vi "MSCOMM.vi"(0 "端口号":string="COM7", 1 "MSComm":refnum<k7>(container), 5 "Send Delay(ms)":string="100", 7 "Send Data":string="AT\r\n", 9 "Data Return":string="OK", 11 "cycle times":string="3") -> (4 "result":bool, 8 "Rec Data":string, 10 "Para":string)   [LabVIEW 2013]
panel:
  out "字符串":string
  out "接收数据长度字节数目":i32
  out "PortOpen":bool
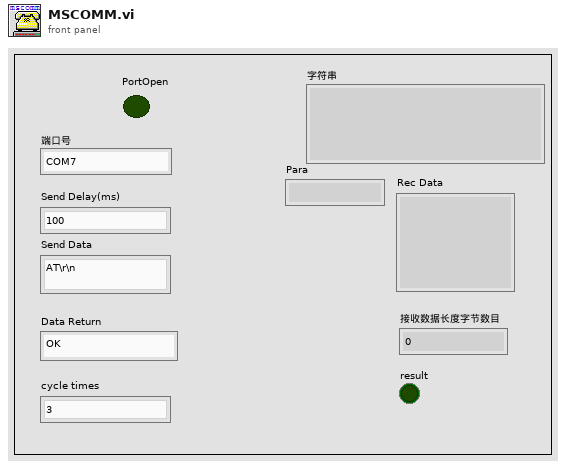
[diagram p1: front panel]
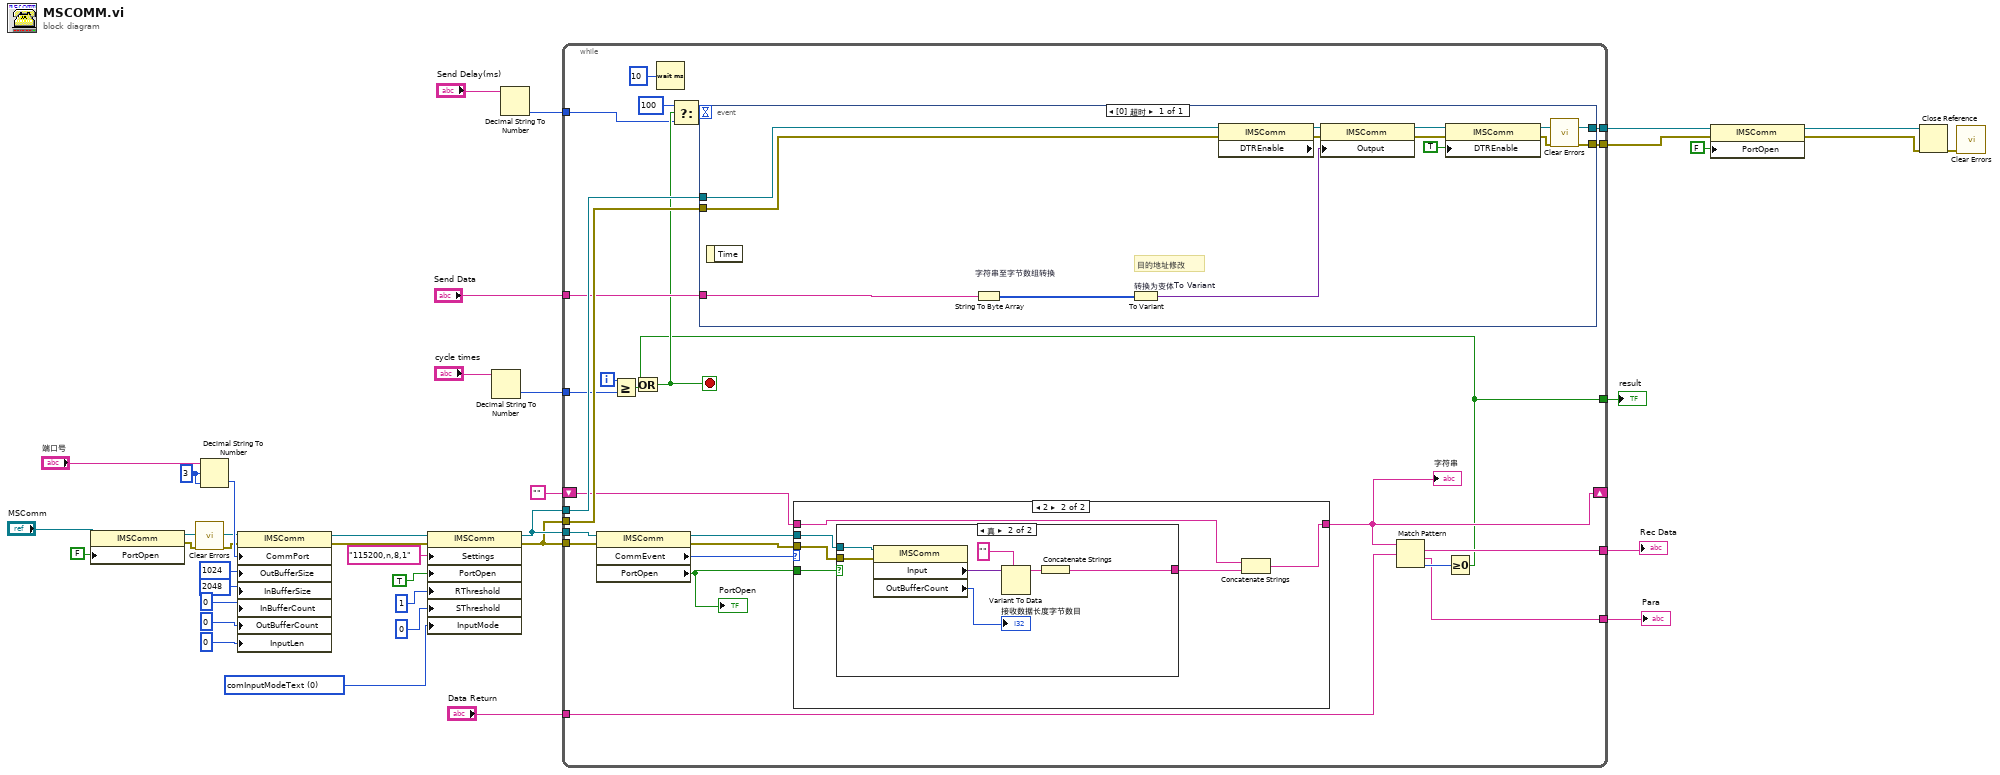
[diagram p0: block diagram]
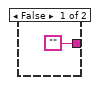
[diagram p3: hidden frame]
diagram:
  w8 = 3 ("偏移量")
  w26 = 0 items=["comInputModeText", "comInputModeBinary"] ("InputMode")
  n1 = property class="IMSComm"(reference="MSComm", "PortOpen"=FALSE) -> (reference out=w6:refnum<k7>, error out=w5:errorcluster)  [unwired: 1 in]
  n2 = call <vilib>:"Clear Errors.vi"("error in (no error)"=w5) -> ("error out"=w4:errorcluster)  [unwired: 6 in]
  n3 = Decimal String To Number(string="端口号", offset=w8, default (0L)=w8) -> (number=w17:i32)  [unwired: 1 out]
  n4 = property class="IMSComm"(reference=w6, error in=w4, "CommPort"=w17, "OutBufferSize"=i16 1024, "InBufferSize"=i16 2048, "InBufferCount"=i16 0, "OutBufferCount"=i16 0, "InputLen"=i16 0) -> (reference out=w25:refnum<k7>, error out=w24:errorcluster)
  n5 = property class="IMSComm"(reference=w25, error in=w24, "Settings"="115200,n,8,1", "PortOpen"=TRUE, "RThreshold"=1, "SThreshold"=0, "InputMode"=w26) -> (reference out=w34:refnum<k7>, error out=w33:errorcluster)
  n6 = Decimal String To Number(string="cycle times") -> (number=w15:i32)  [unwired: 2 in, 1 out]
  n7 = Decimal String To Number(string="Send Delay(ms)") -> (number=w20:i32)  [unwired: 2 in, 1 out]
  n8 = while {
    tunnel: w33 -> [w64]
    tunnel: w34 -> [w63]
    tunnel: w34 -> [w62]
    shift-right: [w54] -> _
    shift-left: "" -> [w61]
    tunnel: w33 -> [w57]
    tunnel: "Data Return" -> [w53]
    tunnel: [w51] -> w22
    tunnel: "Send Data" -> [w50]
    tunnel: w20 -> [w45]
    tunnel: w15 -> [w48]
    tunnel: [w42] -> w14
    tunnel: [w41] -> w13
    tunnel: [w40] -> w2
    tunnel: [w39] -> w1
    i -> [w49]
    stop <- w46 stop-if-true
    n9 = property class="IMSComm"(reference=w62, error in=w57) -> (reference out=w59:refnum<k7>, error out=w55:errorcluster, "CommEvent"=w60:i16, "PortOpen"=w56:bool)
    "PortOpen" <- w56
    n10 = Greater Or Equal?(x=w49, y=w48) -> (x >= y?=w47:bool)
    n11 = Wait (ms)(milliseconds to wait=10) -> ()  [unwired: 1 out]
    n12 = case shown="2" w60 {
      tunnel: w59 -> [_ w71]
      tunnel: w56 -> [_ w67]
      tunnel: w61 -> [w65 w70]
      tunnel: [w65 w69] -> w54
      tunnel: w55 -> [_ w66]
      frame 0, Default {
      }
      frame 2 {
        n13 = case shown="真" w67 {
          tunnel: w71 -> [_ w79]
          tunnel: ["" w74] -> w68
          tunnel: w66 -> [_ w73]
          frame False {
          }
          frame True {
            n14 = property class="IMSComm"(reference=w79, error in=w73) -> ("Input"=w78:variant, "OutBufferCount"=→"接收数据长度字节数目":i16)  [unwired: 2 out]
            n15 = Variant To Data(type="", Variant=w78) -> (data=w75:string)  [unwired: 1 in, 1 out]
            n16 = Concatenate Strings(w75) -> (w74:string)
          }
        }
        n17 = Concatenate Strings(w70, w68) -> (w69:string)
      }
    }
    "字符串" <- w54
    n18 = Match Pattern(string=w54, regular expression=w53) -> (match substring=w51:string, after substring=w39:string, offset past match=w52:i32)  [unwired: 1 in, 1 out]
    n19 = Greater Or Equal To 0?(x=w52) -> (x >= 0?=w40:bool)
    n20 = Or(x=w40, y=w47) -> (x .or. y?=w46:bool)
    n21 = Select(t=100, s=w46, f=w45) -> (s? t:f=w43:i32)
    n22 = event shown="[0] 超时" {
      selector: _ -> [_]
      dyn-events: _ -> [_]
      timeout: w43 -> [_]
      tunnel: w64 -> [w86]
      tunnel: w63 -> [w85]
      tunnel: w50 -> [w83]
      tunnel: [w81] -> w42
      tunnel: [w80] -> w41
      event Timeout {
        # "目的地址修改"
        n23 = event-data() -> ()  [unwired: 2 out]
        n24 = String To Byte Array "字符串至字节数组转换"(string=w83) -> (unsigned byte array=w87:u8[])
        n25 = To Variant "转换为变体To Variant"(anything=w87) -> (Variant=w88:variant)
        n26 = property class="IMSComm" props=["DTREnable"](reference=w85, error in=w86) -> (reference out=w92:refnum<k7>, error out=w91:errorcluster)  [unwired: 1 out]
        n27 = property class="IMSComm"(reference=w92, error in=w91, "Output"=w88) -> (reference out=w90:refnum<k7>, error out=w89:errorcluster)
        n28 = property class="IMSComm"(reference=w90, error in=w89, "DTREnable"=TRUE) -> (reference out=w80:refnum<k7>, error out=w82:errorcluster)
        n29 = call <vilib>:"Clear Errors.vi"("error in (no error)"=w82) -> ("error out"=w81:errorcluster)  [unwired: 6 in]
      }
    }
  }
  "Rec Data" <- w22
  "result" <- w2
  "Para" <- w1
  n30 = property class="IMSComm"(reference=w13, error in=w14, "PortOpen"=FALSE) -> (reference out=w12:refnum<k7>, error out=w11:errorcluster)
  n31 = Close Reference(reference=w12, error in (no error)=w11) -> (error out=w9:errorcluster)
  n32 = call <vilib>:"Clear Errors.vi"("error in (no error)"=w9) -> ()  [unwired: 6 in, 1 out]
